vi "StartExperiment.vi"(8 "error in (no error)":errorcluster, 10 "channel":u8, 11 "deviceName":string) -> (0 "error out":errorcluster, 3 "Success":bool)   [LabVIEW 2018]
doc: "EXPORT bool AisStartExperiment(const char* deviceName, uint8_t channel);"
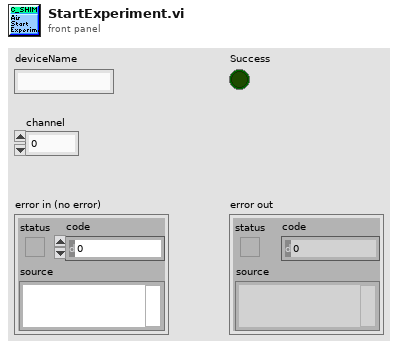
[diagram p1: front panel]
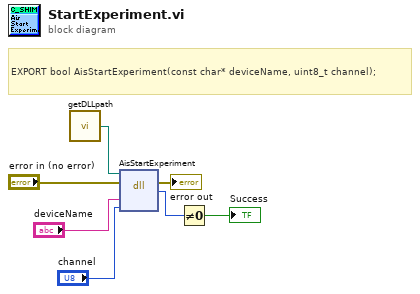
[diagram p0: block diagram]
diagram:
  # "EXPORT bool AisStartExperiment(const char* deviceName, uint8_t channel);"
  n1 = call "getDLLpath.vi"() -> ("DLL_Path"=w1:path)
  n2 = dll-call lib="?" fn="AisStartExperiment"(path in=w1, error in="error in (no error)", "deviceName"="deviceName", "channel"="channel") -> (error out=→"error out":errorcluster, "return type"=w6:u8)  [unwired: 3 in, 1 out]
  n3 = Not Equal To 0?(x=w6) -> (x != 0?=→"Success":bool)
